vi "Set Selection by Start and Length.vi"(8 "error in (no error)":errorcluster caption="错误输入（无错误）", 9 "SelectionLength":i32, 10 "SelectionStart":i32, 11 "RichText 输入":refnum<class "RichText.lvclass"> caption="DNL_LabVIEW Object in") -> (0 "error out":errorcluster caption="错误输出", 3 "RichText 输出":refnum<class "RichText.lvclass"> caption="DNL_LabVIEW Object out")   [LabVIEW 2012, in "RichText.lvclass"]
uses:
  RichText.lvclass
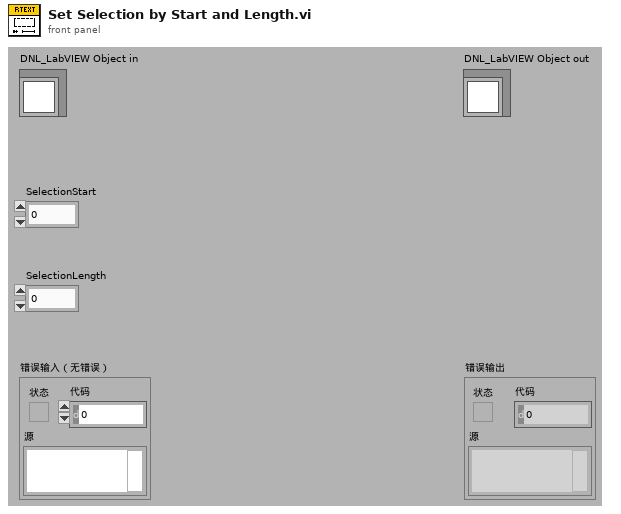
[diagram p1: front panel]
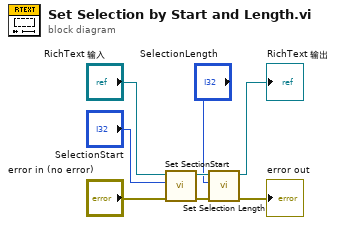
[diagram p0: block diagram]
diagram:
  n1 = call "Set SectionStart.vi"("error in (no error)"="error in (no error)", "SelectionStart"="SelectionStart", "RichText 输入"="RichText 输入") -> ("error out"=w5:errorcluster, "RichText 输出"=w7:refnum<class "RichText.lvclass">)  [unwired: 7 in]
  n2 = call "Set Selection Length.vi"("error in (no error)"=w5, "SelectionLength"="SelectionLength", "RichText 输入"=w7) -> ("error out"=→"error out":errorcluster, "RichText 输出"=→"RichText 输出":refnum<class "RichText.lvclass">)  [unwired: 7 in]
